vi "Agilent 2000 3000 X-Series Real Time Eye.vi"() -> ()   [LabVIEW 2015]
doc: "This example shows how to configure real time eye analysis and take measurements.\n\n<b>Note:</b>\nThis example is specific to the 6000-X Series oscilloscopes. These features are not available on other models."
uses:
  <instrlib>/Agilent 2000 3000 X-Series/Agilent 2000 3000 X-Series.lvlib
panel:
  in  "Frequency (1000 Hz)":dbl=10000000.0
  out "Eye Width":dbl
  out "Eye Height":dbl
  in  "Delay (5 s)":i32=5
  out "UI Intervals Folded Into Real-Time Eye":i32
  in  "Real Time Eye Source (1: Channel 1)":i32(ring)=1 items=["Channel 1"=1, "Channel 2"=2, "Channel 3"=3, "Channel 4"=4]
  in  "Enable Real Time Eye Analysis (T: Enable)":bool=TRUE
  in  "Enable Output (F: Disable)":bool=TRUE
  in  "Waveform Generator Number (1: Waveform Generator 1)":i32(ring)=2 items=["Waveform Generator 1"=1, "Waveform Generator 2"=2]
  in  "Function Type (0: Sine)":i32(ring) items=["Sine", "Square", "Ramp", "Pulse", "Noise", "DC", "Sine Cardinal", "Exponential Rise", "Exponential Fall", "Cardiac", "Gaussian Pulse", "Arbitrary"]
  in  "VISA resource name":refnum<visa-resource-name>
  # "(c) 2011-2016 National Instruments.  ALL RIGHTS RESERVED."
  # "Waveform Generator Configuration"
  # "Real Time Eye Configuration"
  # "Real Time Eye Measurements"
  # "Delay for Data Acquisition"
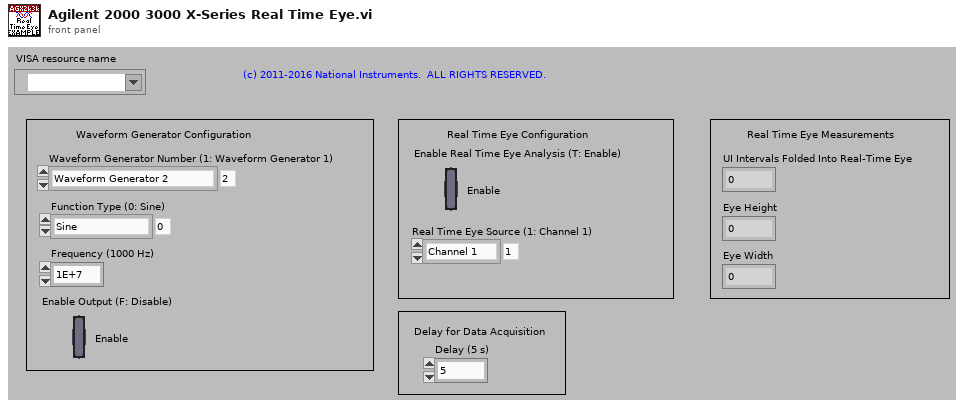
[diagram p1: front panel]
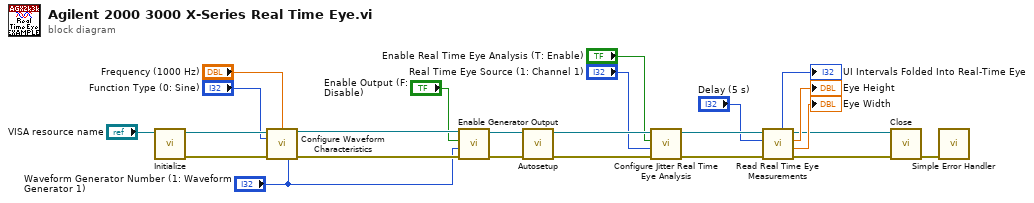
[diagram p0: block diagram]
diagram:
  n1 = call <instrlib>:"Initialize.vi"("VISA resource name"="VISA resource name") -> ("error out"=w21:errorcluster, "VISA resource name out"=w22:refnum<visa-resource-name>)  [unwired: 9 in]
  n2 = call <instrlib>:"Configure Waveform Characteristics.vi"("VISA resource name"=w22, "Frequency (1000 Hz)"="Frequency (1000 Hz)", "Function Type (0: Sine)"="Function Type (0: Sine)", "error in (no error)"=w21, "Waveform Generator Number (1: Waveform Generator 1)"="Waveform Generator Number (1: Waveform Generator 1)") -> ("VISA resource name out"=w20:refnum<visa-resource-name>, "error out"=w19:errorcluster)  [unwired: 9 in]
  n3 = call <instrlib>:"Enable Generator Output.vi"("error in (no error)"=w19, "Waveform Generator Number (1: Waveform Generator 1)"="Waveform Generator Number (1: Waveform Generator 1)", "Enable Output (F: Disable)"="Enable Output (F: Disable)", "VISA resource name"=w20) -> ("error out"=w17:errorcluster, "VISA resource name out"=w18:refnum<visa-resource-name>)  [unwired: 6 in]
  n4 = call <instrlib>:"Autosetup.vi"("error in (no error)"=w17, "VISA resource name"=w18) -> ("error out"=w15:errorcluster, "VISA resource name out"=w16:refnum<visa-resource-name>)  [unwired: 8 in]
  n5 = call <instrlib>:"Configure Jitter Real Time Eye Analysis.vi"("error in (no error)"=w15, "Real Time Eye Source (1: Channel 1)"="Real Time Eye Source (1: Channel 1)", "Enable Real Time Eye Analysis (T: Enable)"="Enable Real Time Eye Analysis (T: Enable)", "VISA resource name"=w16) -> ("error out"=w13:errorcluster, "VISA resource name out"=w14:refnum<visa-resource-name>)  [unwired: 6 in]
  n6 = call <instrlib>:"Read Real Time Eye Measurements.vi"("error in (no error)"=w13, "Delay (5 s)"="Delay (5 s)", "VISA resource name"=w14) -> ("error out"=w1:errorcluster, "Eye Width"=→"Eye Width":dbl, "Eye Height"=→"Eye Height":dbl, "VISA resource name out"=w2:refnum<visa-resource-name>, "UI Intervals Folded Into Real-Time Eye"=→"UI Intervals Folded Into Real-Time Eye":i32)  [unwired: 4 in]
  n7 = call <instrlib>:"Close.vi"("error in (no error)"=w1, "VISA resource name"=w2) -> ("error out"=w24:errorcluster)  [unwired: 9 in]
  n8 = call <vilib>:"Simple Error Handler.vi"("error in (no error)"=w24) -> ()  [unwired: 4 in, 5 out]
